vi "MultiLoop(Notifier).vi"() -> ()   [LabVIEW 2023]
panel:
  out "Waveform Chart 3":dbl(graph)
  out "Waveform Chart 2":dbl(graph)
  in  "Stop Button":bool
  out "Waveform Chart":dbl(graph)
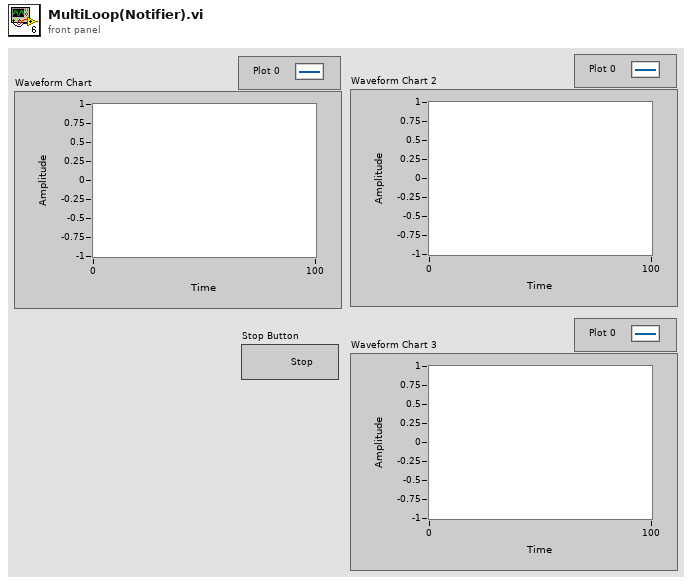
[diagram p1: front panel]
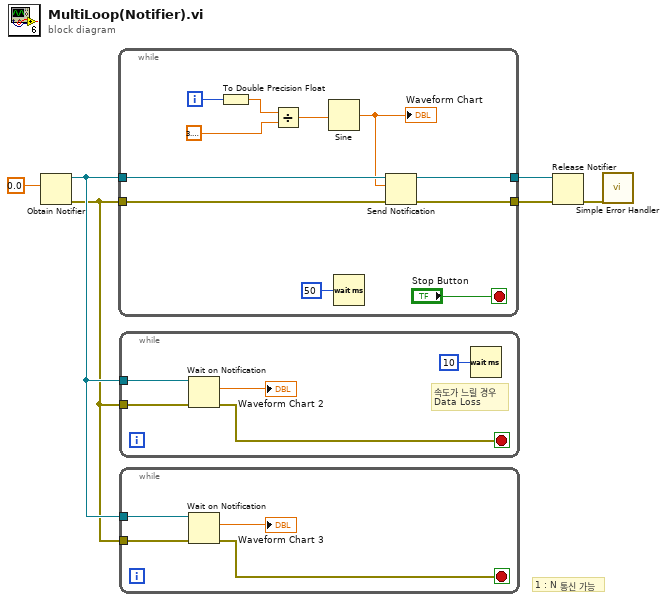
[diagram p0: block diagram]
diagram:
  # "1 : N 통신 가능"
  n1 = Obtain Notifier(notification data type=0.0 ("element data type")) -> (notifier out=w2:refnum<notifier>, error out=w1:errorcluster)  [unwired: 3 in, 1 out]
  n2 = while {
    tunnel: [w11] -> w4
    tunnel: w2 -> [w10]
    tunnel: [w9] -> w5
    tunnel: w1 -> [w7]
    i -> [w17]
    stop <- "Stop Button" stop-if-true
    n3 = To Double Precision Float(number=w17) -> (double precision float=w16:dbl)
    n4 = Divide(x=w16, y=3.141592653589793) -> (x/y=w12:dbl)
    n5 = Sine(x=w12) -> (sin(x)=w8:dbl)
    "Waveform Chart" <- w8
    n6 = Wait (ms)(milliseconds to wait=u32 50) -> ()  [unwired: 1 out]
    n7 = Send Notification(notification=w8, notifier=w10, error in (no error)=w7) -> (notifier out=w9:refnum<notifier>, error out=w11:errorcluster)
  }
  n8 = while {
    tunnel: w2 -> [w21]
    tunnel: w1 -> [w19]
    stop <- w18 stop-if-true
    # "속도가 느릴 경우\nData Loss"
    n9 = Wait on Notification(notifier=w21, error in (no error)=w19) -> (notification=→"Waveform Chart 2":dbl, error out=w18:errorcluster)  [unwired: 2 in, 2 out]
    n10 = Wait (ms)(milliseconds to wait=u32 10) -> ()  [unwired: 1 out]
  }
  n11 = while {
    tunnel: w2 -> [w26]
    tunnel: w1 -> [w24]
    stop <- w23 stop-if-true
    n12 = Wait on Notification(notifier=w26, error in (no error)=w24) -> (notification=→"Waveform Chart 3":dbl, error out=w23:errorcluster)  [unwired: 2 in, 2 out]
  }
  n13 = Release Notifier(notifier=w5, error in (no error)=w4) -> (error out=w3:errorcluster)  [unwired: 1 in, 2 out]
  n14 = call <vilib>:"Simple Error Handler.vi"("error in (no error)"=w3) -> ()  [unwired: 4 in, 5 out]
